vi "InitPerspective.vi"(4 "Far Clipping Plane":sgl, 6 "Near Clipping Plane":sgl, 8 "error in (no error)":errorcluster, 10 "Field of View":sgl, 11 "Render Window in":refnum<class "Render Window.lvclass">) -> (0 "error out":errorcluster, 3 "Render Window out":refnum<class "Render Window.lvclass">)   [LabVIEW 2015, in "Render Window.lvclass"]
uses:
  Render Window.lvclass
  Render Window.lvclass/Render Window.ctl
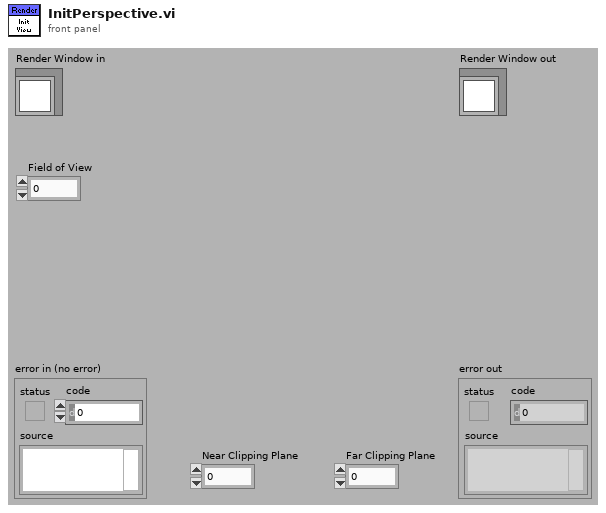
[diagram p1: front panel]
types:
  T1 = typedef "LVRectTypeDef.ctl" = cluster{"Left":i16, "Top":i16, "Right":i16, "Bottom":i16}
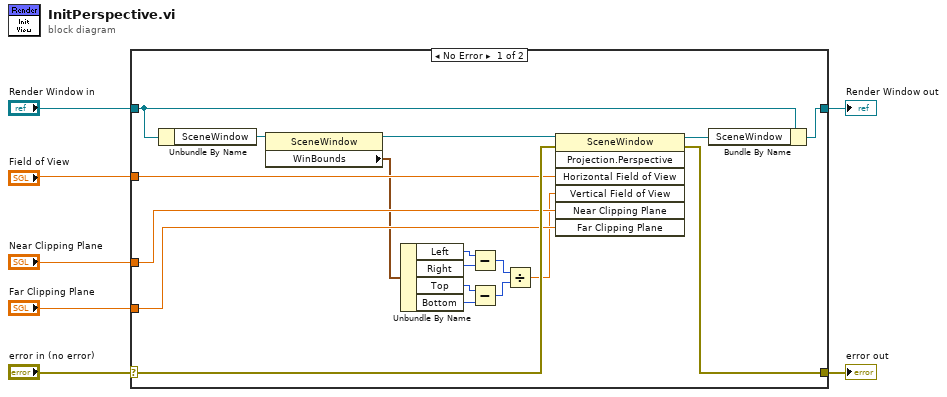
[diagram p0: block diagram]
diagram:
  n1 = case shown="No Error" "error in (no error)" {
    selector: "error in (no error)" -> [w22 w27]
    tunnel: [w21 w27] -> w6
    tunnel: [w23 w26] -> w4
    tunnel: "Render Window in" -> [w24 w26]
    tunnel: "Field of View" -> [w20 _]
    tunnel: "Near Clipping Plane" -> [w19 _]
    tunnel: "Far Clipping Plane" -> [w18 _]
    frame No Error {
      n2 = Unbundle By Name(w24) -> ("SceneWindow"=w16:refnum<vi>)
      n3 = property class="SceneWindow"(reference=w16) -> (reference out=w15:refnum<vi>, "WinBounds"=w17:T1)  [unwired: 1 in, 1 out]
      n4 = Unbundle By Name(w17) -> ("Left"=w13:i16, "Right"=w14:i16, "Top"=w11:i16, "Bottom"=w12:i16)
      n5 = Subtract(x=w13, y=w14) -> (x-y=w9:i16)
      n6 = Subtract(x=w11, y=w12) -> (x-y=w10:i16)
      n7 = Divide(x=w9, y=w10) -> (x/y=w8:dbl)
      n8 = invoke class="SceneWindow" method="Projection.Perspective"(reference=w15, error in=w22, "Horizontal Field of View"=w20, "Vertical Field of View"=w8, "Near Clipping Plane"=w19, "Far Clipping Plane"=w18) -> (reference out=w25:refnum<vi>, error out=w21:errorcluster)  [unwired: 1 in, 5 out]
      n9 = Bundle By Name(cluster=w24, "SceneWindow"=w25) -> (w23:refnum<class "Render Window.lvclass">)
    }
    frame Error {
    }
  }
  "error out" <- w6
  "Render Window out" <- w4
